vi "Read configuration.vi"(8 "error in":errorcluster, 11 "Conversion editor node in":refnum<class "Conversion editor node.lvclass">) -> (0 "error out":errorcluster, 2 "configuration":refnum<class "NISE_CEF_serializable configuration.lvclass">, 3 "Conversion editor node out":refnum<class "Conversion editor node.lvclass">)   [LabVIEW 2017, in "Conversion editor node.lvclass"]
uses:
  Conversion editor node.lvclass
  <vilib>/NI/Configuration Framework/serializable configuration/NISE_CEF_serializable configuration.lvclass
  Conversion editor node.lvclass/Conversion editor node.ctl
  module/configuration/Conversion configuration.lvclass
  C:/Program Files (x86)/National Instruments/LabVIEW 2017/vi.lib/NI/Configuration Framework/serializable configuration/NISE_CEF_serializable configuration.lvclass
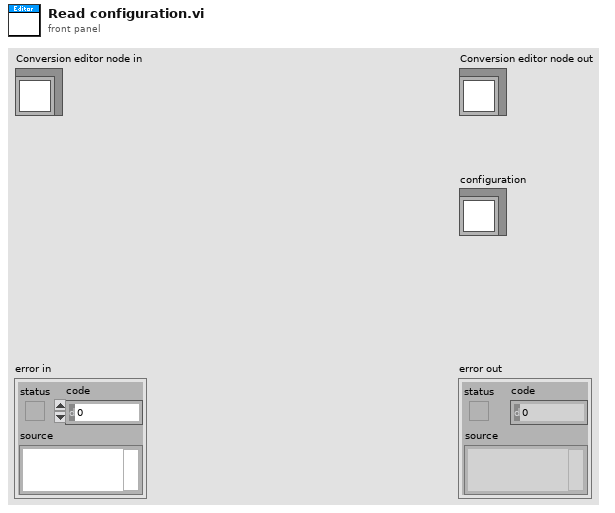
[diagram p1: front panel]
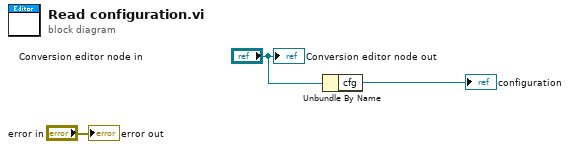
[diagram p0: block diagram]
diagram:
  n1 = Unbundle By Name("Conversion editor node in") -> ("cfg"=→"configuration":refnum<class "Conversion configuration.lvclass">)
  "error out" <- "error in"
  "Conversion editor node out" <- "Conversion editor node in"
